vi "SoftFrontPanel.vi"(8 "error in":errorcluster, 11 "Digitizer Channel":refnum<class "Digitizer Channel.lvclass">) -> (0 "error out":errorcluster, 3 "Digitizer Channel out":refnum<class "Digitizer Channel.lvclass">)   [LabVIEW 2025, in "Digitizer.lvlib" / "Digitizer Channel.lvclass"]
doc: "Copyright 2017 National Instruments Corporation\n\nLicensed under the Apache License, Version 2.0 (the \"License\"); you may not use this file except in compliance with the License. You may obtain a copy of the License at http://www.apache.org/licenses/LICENSE-2.0\nUnless required by applicable law or agreed to in writing, software distributed under the License is distributed on an \"AS IS\" BASIS, WITHOUT WARRANTIES OR CONDITIONS OF ANY KIND, either express or implied. See the License for the specific language governing permissions and limitations under the License."
uses:
  Digitizer Channel.lvclass
  Digitizer Channel.lvclass/Digitizer Channel.ctl
  Digitizer Instrument/Digitizer Instrument.lvclass
  C:/Users/Public/Documents/Sandia National Labs/TSS Plugin/Abstract Engine.lvlibp/Plugin/Abstract/Abstract Instrument/Abstract Instrument.lvclass
  C:/Users/Public/Documents/Sandia National Labs/TSS Plugin/CEF.lvlibp/serializable node/CEF_serializable node.lvclass
  C:/Users/Public/Documents/Sandia National Labs/TSS Plugin/CEF.lvlibp/Node/CEF_Node.lvclass
  C:/Working copy/tss/Plugin/Engines/Digitizer/Digitizer Instrument/Digitizer Instrument.lvclass
  Digitizer Channel configuration/Digitizer Channel configuration.lvclass
  Users/Public/Documents/Sandia National Labs/TSS Plugin/CEF.lvlibp
  Users/Public/Documents/Sandia National Labs/TSS Plugin/Abstract Engine.lvlibp/Plugin/Abstract/Abstract Instrument/Abstract Instrument.lvclass
panel:
  out "Chart Msg":string
  out "Waveform Chart":waveform(dbl)(graph)
  out "Channel":string caption="Channel ::"
  # "Live Value"
  # "V"
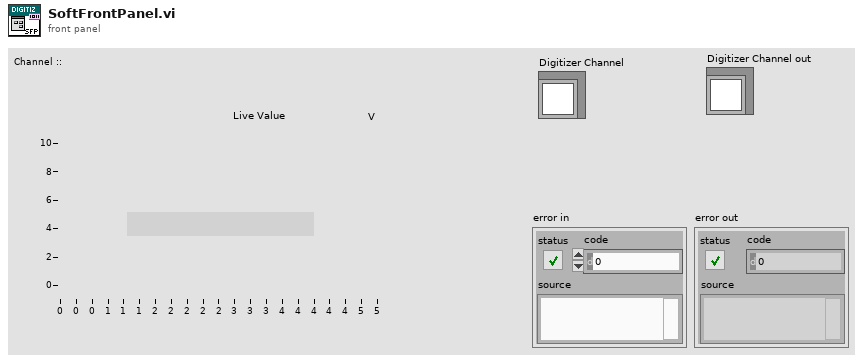
[diagram p1: front panel]
types:
  T1 = enum32{"Invalid", "Default", "Floating", "Floating/Auto-Hide", "Modal"}
  T2 = cluster{"Address":string, "SW Alias":string, "Enabled":bool, "Type":string, "Description":string}
  T3 = typedef "Digitizer.lvlib/Digitizer Instrument.lvclass/Digitizer Dataset.ctl" = cluster{"Channel":string, "Waveform":waveform(dbl)}
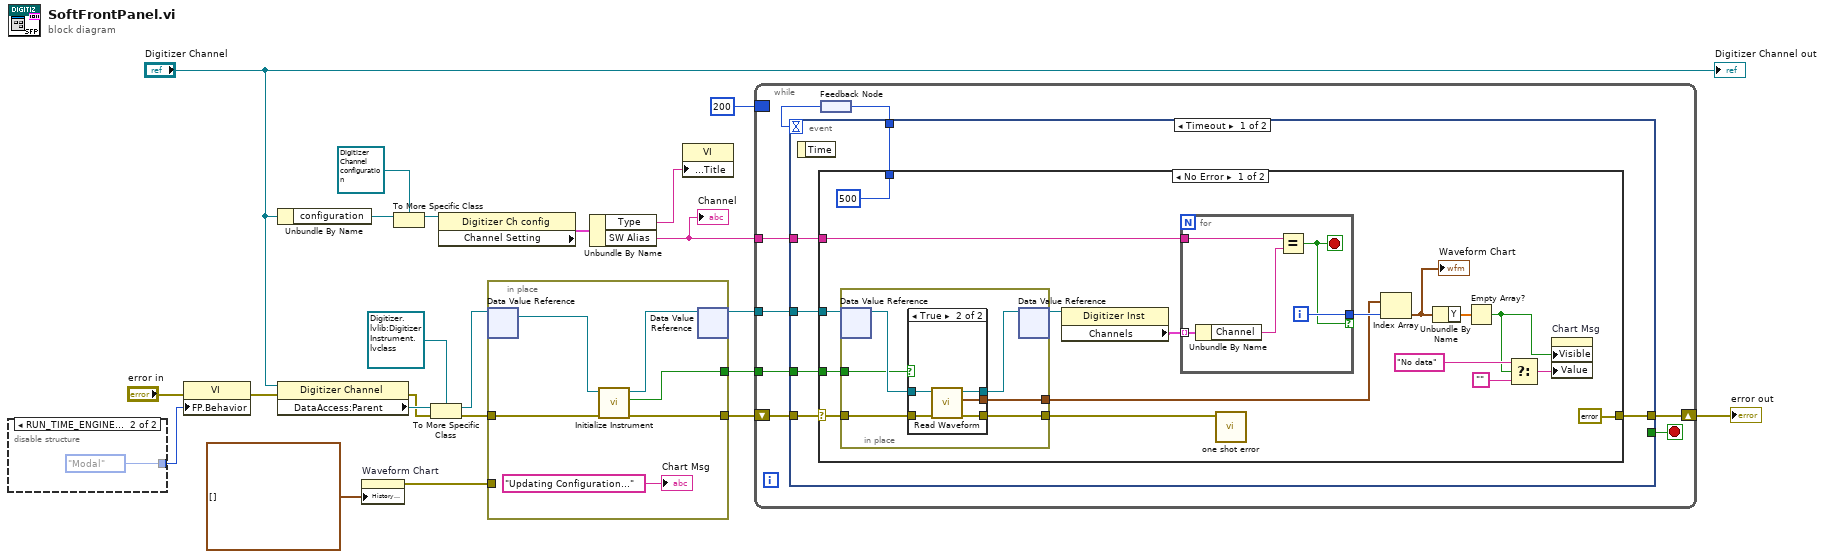
[diagram p0: block diagram]
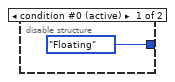
[diagram p2: hidden frame]
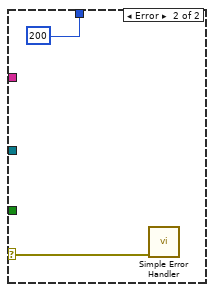
[diagram p4: hidden frame]
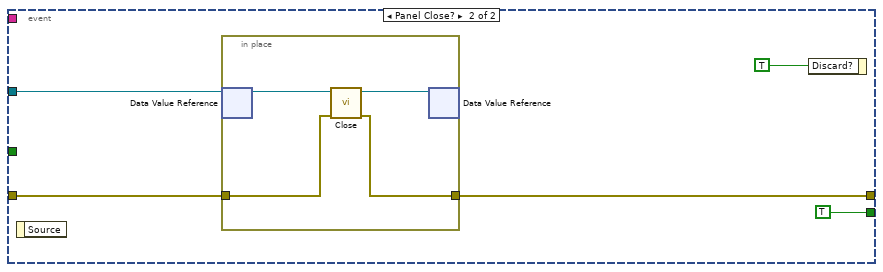
[diagram p5: hidden frame]
diagram:
  n1 = disable-structure shown="RUN_TIME_ENGINE==True" {
    disable-tunnel: [T1."Floating" ("Front Panel Window:Behavior") T1."Modal" ("Front Panel Window:Behavior")] -> w20
    frame condition #0 (active) {
    }
    frame condition #1 {
    }
  }
  n2 = property class="VI"(error in="error in", "FP.Behavior"=w20) -> (error out=w19:errorcluster)  [unwired: 1 in, 1 out]
  n3 = Unbundle By Name("Digitizer Channel") -> ("configuration"=w8:refnum<class "Digitizer Channel configuration.lvclass">)
  n4 = property class="Digitizer Channel"(reference="Digitizer Channel", error in=w19) -> (error out=w16:errorcluster, "DataAccess:Parent"=w17:refnum<data-value>)  [unwired: 1 out]
  n5 = property on="Waveform Chart" class="WFChart (strict)"("History Data"=waveform(dbl)[] []) -> (error out=w6:errorcluster)  [unwired: 2 in, 1 out]
  n6 = To More Specific Class(target class=refnum<class "Digitizer Channel configuration.lvclass"> refnum ("Digitizer.lvlib:Digitizer Channel configuration.lvclass"), reference=w8) -> (specific class reference=w12:refnum<class "Digitizer Channel configuration.lvclass">)  [unwired: 1 in, 1 out]
  n7 = To More Specific Class(target class=refnum<data-value> refnum ("data value reference"), reference=w17, error in=w16) -> (specific class reference=w15:refnum<data-value>, error out=w14:errorcluster)
  n8 = property class="Digitizer Ch config"(reference=w12) -> ("Channel Setting"=w10:T2)  [unwired: 1 in, 2 out]
  n9 = in-place {
    in-place-border: w14 -> [w28]
    in-place-border: [w27] -> w3
    in-place-border: w6 -> [_]
    in-place-border: [w25] -> w5
    # "Initialize the front panel controls when loaded"
    n10 = in-place-dvr #1(w15) -> (w29:refnum<class "Digitizer Instrument.lvclass">)  [unwired: 1 out]
    n11 = call "Initialize Instrument.vi"("error in"=w28, "Abstract Instrument"=w29) -> ("error out"=w27:errorcluster, "Found?"=w25:bool, "Abstract Instrument out"=w26:refnum<class "Digitizer Instrument.lvclass">)  [unwired: 7 in]
    n12 = in-place-dvr #1(w26) -> (w13:refnum<data-value>)  [unwired: 1 out]
    "Chart Msg" <- "Updating Configuration..." ("No data")
  }
  n13 = Unbundle By Name(w10) -> ("Type"=w1:string, "SW Alias"=w2:string)
  "Channel" <- w2
  n14 = property class="VI"("Front Panel.Title"=w1) -> ()  [unwired: 2 in, 2 out]
  n15 = while {
    tunnel: w13 -> [w35]
    tunnel: w2 -> [w34]
    tunnel: w5 -> [w33]
    border: 200 -> [_]
    shift-right: [w36] -> w22
    shift-left: w3 -> [w37]
    stop <- w38 stop-if-true
    n16 = feedback #2() -> (w31:i32)
    n17 = event shown="[0] Timeout" {
      selector: _ -> [_ _]
      dyn-events: _ -> [_ _]
      timeout: w31 -> [_ _]
      tunnel: [_ TRUE] -> w38
      tunnel: [w42 w82] -> w36
      tunnel: w37 -> [w41 w83]
      tunnel: w35 -> [w44 w84]
      tunnel: w34 -> [w43 _]
      tunnel: w33 -> [w40 _]
      tunnel: [w39 _] -> w32
      event Timeout {
        n18 = event-data() -> ()  [unwired: 1 in, 1 out]
        n19 = case shown="No Error" w41 {
          selector: w41 -> [w49 w81]
          tunnel: w44 -> [w61 _]
          tunnel: w43 -> [w58 _]
          tunnel: [errorcluster {"status"=FALSE, "code"=0, "source"=""} ("error out") _] -> w42
          tunnel: w40 -> [w46 _]
          tunnel: [500 200] -> w39
          frame No Error {
            n20 = in-place {
              in-place-border: w49 -> [w69]
              in-place-border: [w71] -> w53
              in-place-border: [w70] -> w47
              in-place-border: w46 -> [w67]
              # "Initialize the front panel controls when loaded"
              n21 = in-place-dvr #3(w61) -> (w68:refnum<class "Digitizer Instrument.lvclass">)  [unwired: 1 out]
              n22 = case shown="True" w67 {
                tunnel: [w73 w79] -> w72
                tunnel: [_ w78] -> w71
                tunnel: [w74 w77] -> w70
                tunnel: w69 -> [w74 w76]
                tunnel: w68 -> [w73 w75]
                frame False {
                }
                frame True {
                  n23 = call-dynamic "Read Waveform.vi"("error in (no error)"=w76, "Digitizer Instrument"=w75) -> ("error out"=w77:errorcluster, "Waveforms"=w78:waveform(dbl)[], "Digitizer Instrument out"=w79:refnum<class "Digitizer Instrument.lvclass">)  [unwired: 7 in]
                }
              }
              n24 = in-place-dvr #3(w72) -> (w59:refnum<data-value>)  [unwired: 1 out]
            }
            n25 = property class="Digitizer Inst"(reference=w59) -> ("Channels"=w60:T3[])  [unwired: 1 in, 2 out]
            n26 = for {
              tunnel: w60 -> [w62] mode=indexing
              tunnel: w58 -> [w66]
              tunnel: [w64] -> w57 if=w63
              i -> [w64]
              stop <- w63 stop-if-true
              n27 = Unbundle By Name(w62) -> ("Channel"=w65:string)
              n28 = Equal?(x=w66, y=w65) -> (x = y?=w63:bool)
            }
            n29 = call "one shot error.vi"("error in"=w47) -> ()  [unwired: 11 in]
            n30 = Index Array(array=w53, index=w57) -> (element=w52:waveform(dbl))
            "Waveform Chart" <- w52
            n31 = Unbundle By Name(w52) -> ("Y"=w54:dbl[])
            n32 = Empty Array?(array=w54) -> (empty?=w50:bool)
            n33 = Select(t="No data" ("No data"), s=w50, f="") -> (s? t:f=w51:string)
            n34 = property on="Chart Msg" class="Str"("Visible"=w50, "Value"=w51) -> ()  [unwired: 2 in, 2 out]
          }
          frame Error {
            n35 = call <vilib>:"Simple Error Handler.vi"("error in (no error)"=w81) -> ()  [unwired: 4 in, 5 out]
          }
        }
      }
      event Panel Close? {
        n36 = event-data() -> ()  [unwired: 1 in, 1 out]
        n37 = in-place {
          in-place-border: w83 -> [w88]
          in-place-border: [w87] -> w82
          # "Initialize the front panel controls when loaded"
          n38 = in-place-dvr #4(w84) -> (w90:refnum<class "Digitizer Instrument.lvclass">)  [unwired: 1 out]
          n39 = call-dynamic "Close.vi"("error in (no error)"=w88, "Abstract Instrument in"=w90) -> ("error out"=w87:errorcluster, "Abstract Instrument out"=w89:refnum<class "Digitizer Instrument.lvclass">)  [unwired: 8 in]
          n40 = in-place-dvr #4(w89) -> ()  [unwired: 2 out]
        }
        n41 = event-data("Discard?"=TRUE) -> ()  [unwired: 1 in, 1 out]
      }
    }
    n42 = feedback-in #2(w32) -> ()
  }
  "error out" <- w22
  "Digitizer Channel out" <- "Digitizer Channel"
